vi "MPExxx_set_ext_ctrl.vi"(2 "error in (no error)":errorcluster, 3 "External Control":bool, 4 "VISA session":refnum<visa-resource-name>) -> (0 "error out":errorcluster, 1 "dup VISA session":refnum<visa-resource-name>)   [LabVIEW 2012]
doc: "This VI form enables or disables the external inputs for start, stop, arm, and clear."
panel:
  # "MAGNA-POWER"
  # "Electronics"
  # "ON"
  # "OFF"
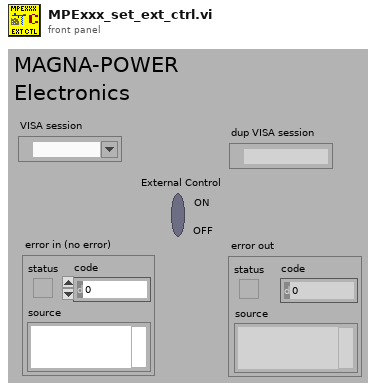
[diagram p1: front panel]
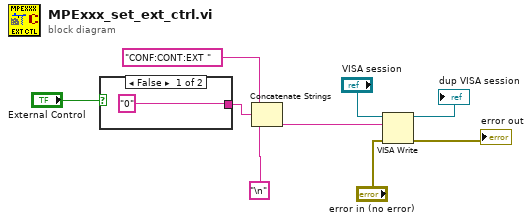
[diagram p0: block diagram]
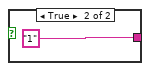
[diagram p2: hidden frame]
diagram:
  n1 = case shown="False" "External Control" {
    tunnel: ["0" "1"] -> w6
    frame False {
    }
    frame True {
    }
  }
  n2 = Concatenate Strings("CONF:CONT:EXT ", w6, "\n") -> (w8:string)
  n3 = VISA Write(VISA resource name="VISA session", write buffer=w8, error in (no error)="error in (no error)") -> (VISA resource name out=→"dup VISA session":refnum<visa-resource-name>, error out=→"error out":errorcluster)  [unwired: 1 out]
